vi "Save HW as XML.vi"(7 "New File":bool, 8 "error in (no error)":errorcluster, 10 "Path":path, 11 "Hardware Settings.lvclass":refnum<class "Hardware Settings.lvclass">) -> (0 "error out":errorcluster)   [LabVIEW 2017, in "Hardware Settings.lvclass"]
uses:
  Hardware Settings.lvclass
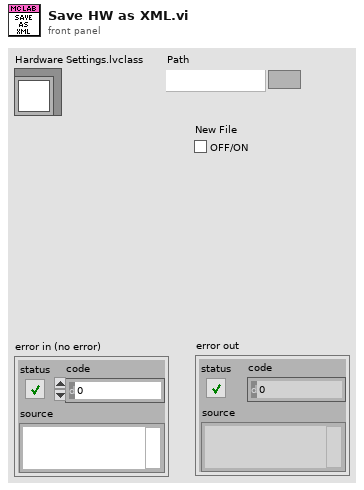
[diagram p1: front panel]
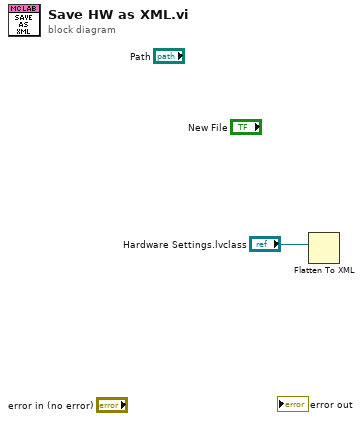
[diagram p0: block diagram]
diagram:
  n1 = Flatten To XML(anything="Hardware Settings.lvclass") -> ()  [unwired: 1 out]
